vi "DecodeCinematics.vi"(8 "error in":errorcluster, 9 "Array":u8[](array[numeric]) format="%02x") -> (0 "error out":errorcluster, 1 "array w/ subset deleted":u8[](array[numeric]), 3 "Cinematics":T1)   [LabVIEW 2017]
panel:
  in  "Cinematics":T1
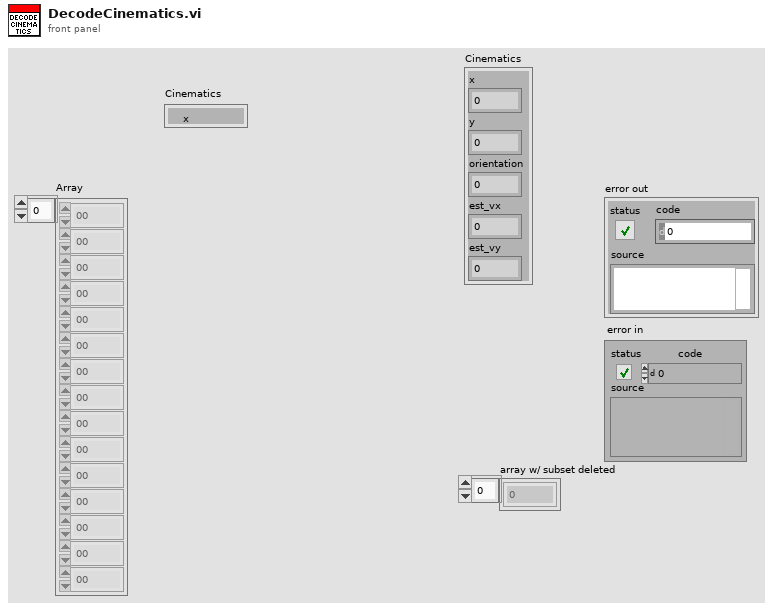
[diagram p1: front panel]
types:
  T1 = cluster{"x":dbl, "y":dbl, "orientation":dbl, "est_vx":dbl, "est_vy":dbl}
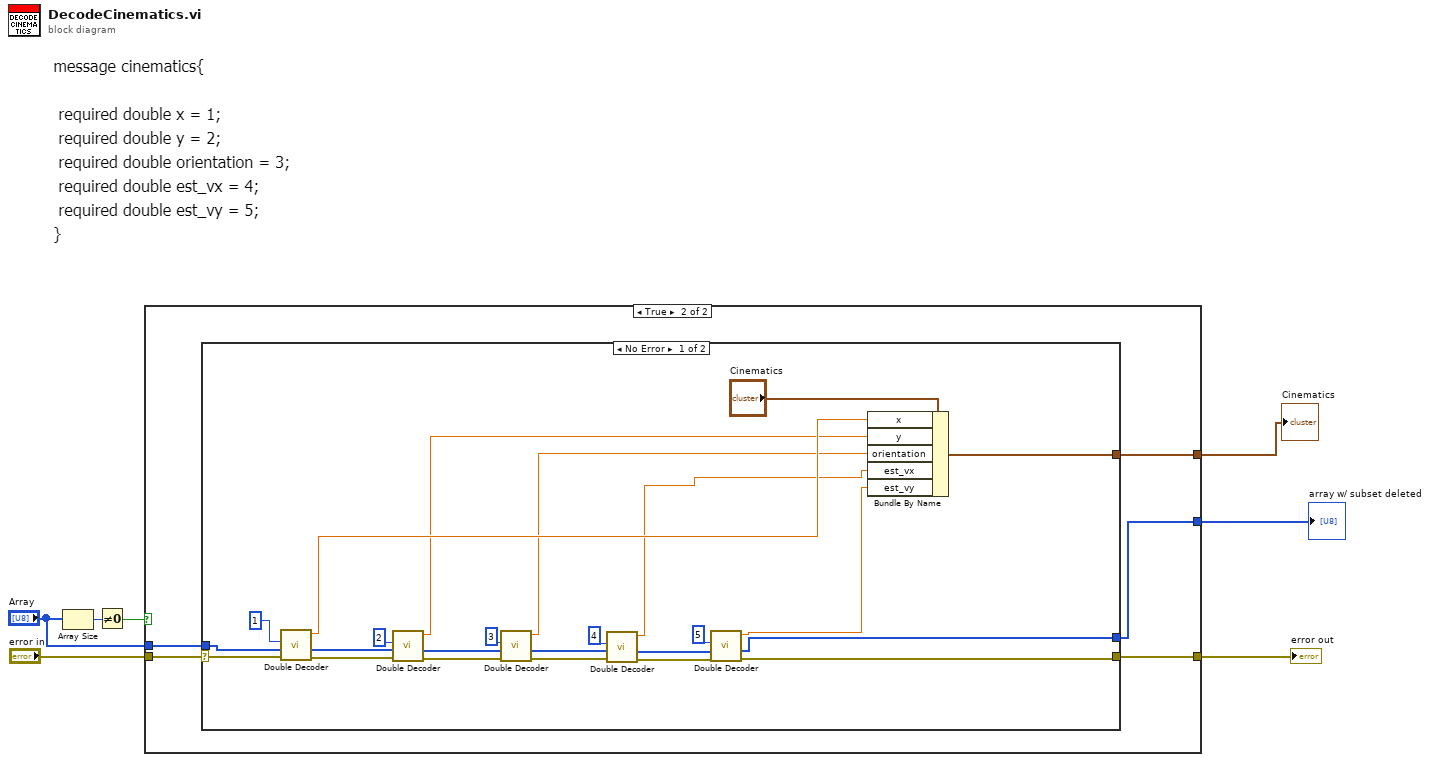
[diagram p0: block diagram]
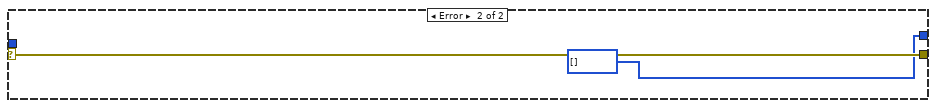
[diagram p3: hidden frame]
diagram:
  n1 = Array Size(array="Array") -> (size(s)=w5:i32)
  n2 = Not Equal To 0?(x=w5) -> (x != 0?=w3:bool)
  n3 = case shown="True" w3 {
    tunnel: "error in" -> [_ w12]
    tunnel: "Array" -> [_ w11]
    tunnel: [_ w10] -> w4
    tunnel: [_ w9] -> w2
    tunnel: [_ w8] -> w1
    frame False {
    }
    frame True {
      n4 = case shown="No Error" w12 {
        selector: w12 -> [w33 w38]
        tunnel: [w21 w38] -> w10
        tunnel: [w20 u8[] [] ("array w/ subset deleted")] -> w9
        tunnel: w11 -> [w34 _]
        tunnel: [w13 _] -> w8
        frame No Error {
          n5 = call "Double Decoder.vi"("error in (no error)"=w33, "Array"=w34, "Key"=1) -> ("error out"=w31:errorcluster, "array w/ subset deleted"=w32:u8[], "Double"=w18:dbl)  [unwired: 5 in, 1 out]
          n6 = call "Double Decoder.vi"("error in (no error)"=w31, "Array"=w32, "Key"=2) -> ("error out"=w36:errorcluster, "array w/ subset deleted"=w35:u8[], "Double"=w17:dbl)  [unwired: 5 in, 1 out]
          n7 = call "Double Decoder.vi"("error in (no error)"=w36, "Array"=w35, "Key"=3) -> ("error out"=w29:errorcluster, "array w/ subset deleted"=w30:u8[], "Double"=w16:dbl)  [unwired: 5 in, 1 out]
          n8 = call "Double Decoder.vi"("error in (no error)"=w29, "Array"=w30, "Key"=4) -> ("error out"=w27:errorcluster, "array w/ subset deleted"=w28:u8[], "Double"=w15:dbl)  [unwired: 5 in, 1 out]
          n9 = call "Double Decoder.vi"("error in (no error)"=w27, "Array"=w28, "Key"=5) -> ("error out"=w21:errorcluster, "array w/ subset deleted"=w20:u8[], "Double"=w14:dbl)  [unwired: 5 in, 1 out]
          n10 = Bundle By Name(cluster="Cinematics", "x"=w18, "y"=w17, "orientation"=w16, "est_vx"=w15, "est_vy"=w14) -> (w13:T1)
        }
        frame Error {
        }
      }
    }
  }
  "error out" <- w4
  "array w/ subset deleted" <- w2
  "Cinematics" <- w1
